vi "your-code-here.vi"(11 "data in":waveform(dbl)[](array[waveform])) -> (3 "data out":waveform(dbl)[](array[waveform]))   [LabVIEW 2024]
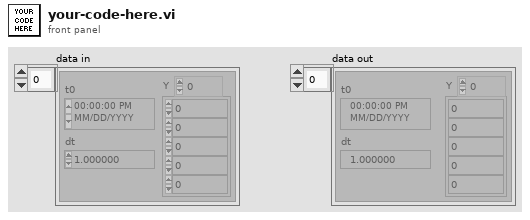
[diagram p1: front panel]
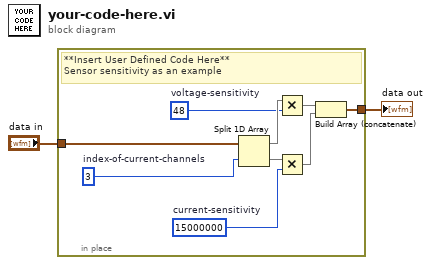
[diagram p0: block diagram]
diagram:
  n1 = in-place {
    in-place-border: "data in" -> [w11]
    in-place-border: [w3] -> w1
    w7 = u64 15000000  # current-sensitivity
    w8 = u64 48  # voltage-sensitivity
    w10 = 3  # index-of-current-channels
    # "**Insert User Defined Code Here**\nSensor sensitivity as an example"
    n2 = Split 1D Array(array=w11, index=w10) -> (first subarray=w9:waveform(dbl)[], second subarray=w6:waveform(dbl)[])
    n3 = Multiply(x=w9, y=w8) -> (x*y=w5:waveform(dbl)[])
    n4 = Multiply(x=w6, y=w7) -> (x*y=w4:waveform(dbl)[])
    n5 = Build Array (concatenate)(w5, w4) -> (w3:waveform(dbl)[])
  }
  "data out" <- w1
